vi "Read NI Configuration File.vi"() -> (0 "Serial Numbers Found":bool, 5 "NI1":dbl, 7 "NI2":dbl)   [LabVIEW 2017]
uses:
  <vilib>/Utility/config.llb/Read Key (I32).vi
  <vilib>/Utility/config.llb/NI_LVConfig.lvlib
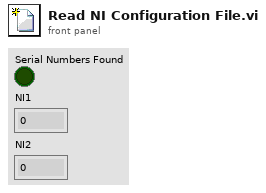
[diagram p1: front panel]
types:
  T1 = typedef "NI_LVConfig.lvlib/Config Data RefNum.ctl" = refnum<k1>
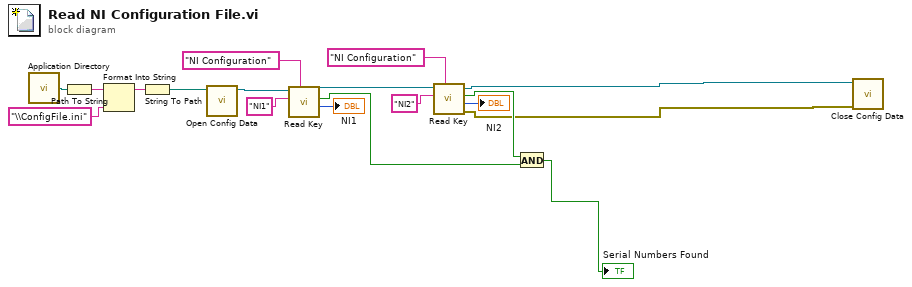
[diagram p0: block diagram]
diagram:
  n1 = call <vilib>:"Application Directory.vi"() -> ("Application Directory"=w18:path)
  n2 = Path To String(path=w18) -> (string=w17:string)
  n3 = Format Into String(initial string=w17, "\\ConfigFile.ini" ("string")) -> (resulting string=w15:string)  [unwired: 2 in, 1 out]
  n4 = String To Path(string=w15) -> (path=w14:path)
  n5 = call <vilib>:"Open Config Data.vi"("configuration file path"=w14) -> ("refnum"=w13:T1)  [unwired: 8 in, 2 out]
  n6 = call-poly <vilib>:"Read Key.vi"("section"="NI Configuration", "key"="NI1", "refnum"=w13) -> ("value"=→"NI1":i32, "found?"=w5:bool, "refnum out"=w9:T1)  [unwired: 5 in, 1 out]
  n7 = call-poly <vilib>:"Read Key.vi"("section"="NI Configuration", "key"="NI2", "refnum"=w9) -> ("error out"=w1:errorcluster, "value"=→"NI2":i32, "found?"=w6:bool, "refnum out"=w2:T1)  [unwired: 5 in]
  n8 = And(x=w6, y=w5) -> (x .and. y?=→"Serial Numbers Found":bool)
  n9 = call <vilib>:"Close Config Data.vi"("error in (no error)"=w1, "refnum"=w2) -> ()  [unwired: 8 in, 2 out]
